vi "update y Scale colors for each plot.vi"(11 "WaveformChart in":refnum<vi>) -> ()   [LabVIEW 2016]
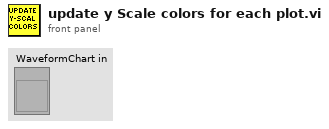
[diagram p1: front panel]
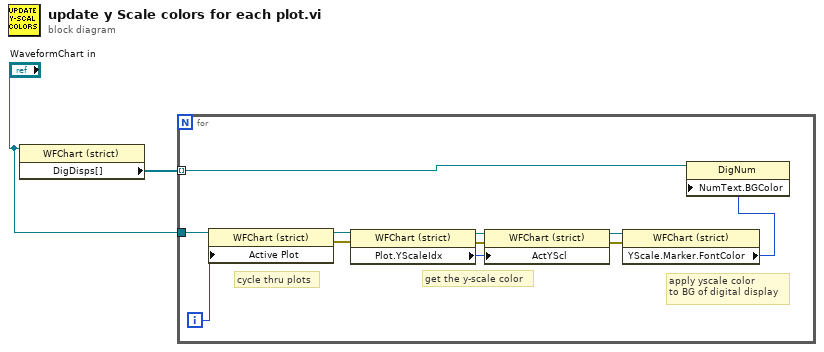
[diagram p0: block diagram]
diagram:
  n1 = property class="WFChart (strict)"(reference="WaveformChart in") -> ("DigDisps[]"=w1:refnum<vi>[])  [unwired: 1 in, 2 out]
  n2 = for {
    tunnel: w1 -> [w13] mode=indexing
    tunnel: "WaveformChart in" -> [w11]
    i -> [w12]
    # "apply yscale color\nto BG of digital display"
    # "get the y-scale color"
    # "cycle thru plots"
    n3 = property class="WFChart (strict)"(reference=w11, "Active Plot"=w12) -> (reference out=w9:refnum<vi>, error out=w10:errorcluster)  [unwired: 1 in]
    n4 = property class="WFChart (strict)"(reference=w9, error in=w10) -> (reference out=w8:refnum<vi>, error out=w7:errorcluster, "Plot.YScaleIdx"=w6:u32)
    n5 = property class="WFChart (strict)"(reference=w8, error in=w7, "ActYScl"=w6) -> (reference out=w5:refnum<vi>, error out=w4:errorcluster)
    n6 = property class="WFChart (strict)"(reference=w5, error in=w4) -> ("YScale.Marker.FontColor"=w3:u32)  [unwired: 2 out]
    n7 = property class="DigNum"(reference=w13, "NumText.BGColor"=w3) -> ()  [unwired: 1 in, 2 out]
  }
